vi "Draw Estimated Pose Covariance.vi"(10 "State Uncertainty":T1, 11 "Estimated State":T1) -> (3 "Covariance Ellipses":cluster{dbl[], dbl[]}[](graph))   [LabVIEW 2020]
uses:
  <vilib>/Analysis/Matrix/Datatypes/RealMatrix.ctl
  <vilib>/Analysis/baseanly.llb/Real A x B.vi
  <vilib>/Analysis/baseanly.llb/A x Vector.vi
  <vilib>/Analysis/7linalg.llb/Real SVD Decomposition.vi
  <vilib>/Analysis/Matrix/Numeric/Conversions/Matrix To Array - RM.vi
  <vilib>/Analysis/NI_AALPro.lvlib
  <vilib>/Analysis/NI_AALBase.lvlib
  <vilib>/Analysis/Matrix/NI_Matrix.lvlib
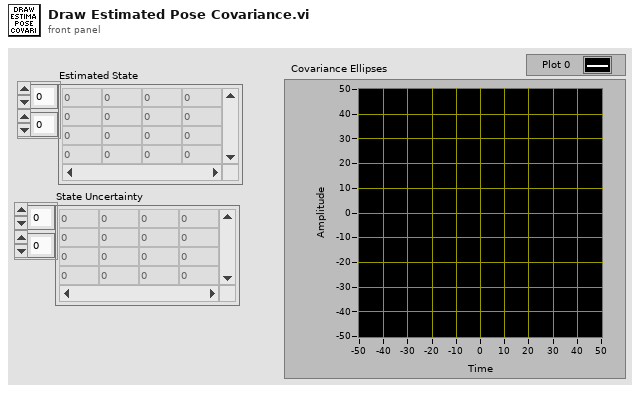
[diagram p1: front panel]
types:
  T1 = typedef "NI_Matrix.lvlib/RealMatrix.ctl" = dbl[][]
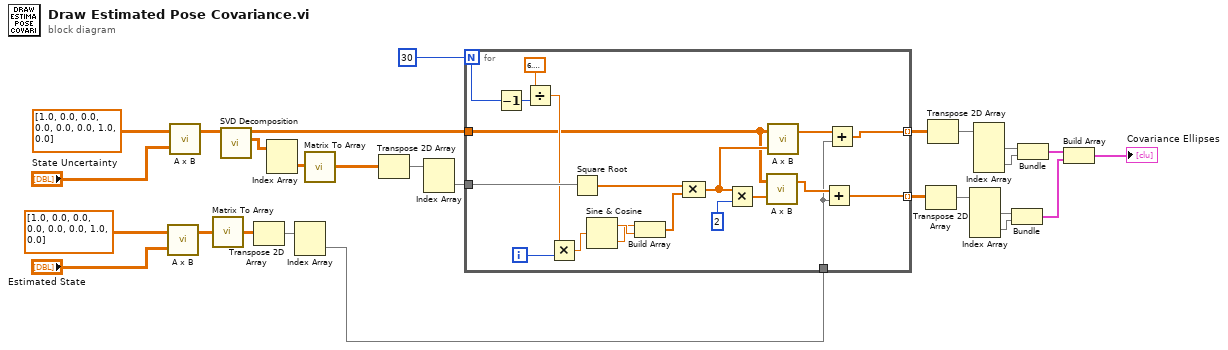
[diagram p0: block diagram]
diagram:
  n1 = call-poly <vilib>:"A x B.vi"("B"="Estimated State", "A"=T1 [[1.0, 0.0, 0.0, 0.0], [0.0, 0.0, 1.0, 0.0]] ("Initial Control Input")) -> ("A x B"=w4:T1)  [unwired: 1 out]
  n2 = call-poly <vilib>:"A x B.vi"("B"="State Uncertainty", "A"=T1 [[1.0, 0.0, 0.0, 0.0], [0.0, 0.0, 1.0, 0.0]] ("Initial Control Input")) -> ("A x B"=w23:T1)  [unwired: 1 out]
  n3 = call-poly <vilib>:"Matrix To Array.vi"("Real Matrix"=w4) -> ("Real 2D Array"=w3:dbl[][])
  n4 = call-poly <vilib>:"SVD Decomposition.vi"("A"=w23) -> ("Matrix S"=w25:T1, "Matrix U"=w27:T1)  [unwired: 6 in, 3 out]
  n5 = Transpose 2D Array(2D array=w3) -> (transposed array=w2:dbl[][])
  n6 = Index Array(array=w25) -> (element=w22:T1)  [unwired: 2 in]
  n7 = Index Array(array=w2) -> (element=w1:dbl[])  [unwired: 2 in]
  n8 = call-poly <vilib>:"Matrix To Array.vi"("Real Matrix"=w22) -> ("Real 2D Array"=w19:dbl[][])
  n9 = Transpose 2D Array(2D array=w19) -> (transposed array=w20:dbl[][])
  n10 = Index Array(array=w20) -> (element=w21:dbl[])  [unwired: 2 in]
  n11 = for {
    N: 30 -> [w37]
    tunnel: w27 -> [w33]
    tunnel: w21 -> [w47]
    tunnel: [w31] -> w18 mode=indexing
    tunnel: [w29] -> w14 mode=indexing
    tunnel: w1 -> [w28]
    i -> [w45]
    n12 = Decrement(x=w37) -> (x-1=w38:i32)
    n13 = Divide(x=6.283185307179586, y=w38) -> (x/y=w44:dbl)
    n14 = Multiply(x=w44, y=w45) -> (x*y=w43:dbl)
    n15 = Square Root(x=w47) -> (sqrt(x)=w40:dbl[])
    n16 = Sine & Cosine(0:w43) -> (1:w42:dbl, 2:w41:dbl)
    n17 = Build Array(w41, w42) -> (w39:dbl[])
    n18 = Compound Arithmetic op=MULTIPLY(w40, w39) -> (w36:dbl[])
    n19 = Multiply(x=w36, y=2) -> (x*y=w34:dbl[])
    n20 = call-poly <vilib>:"A x B.vi"("Vector"=w34, "A"=w33) -> ("A x Vector"=w30:dbl[])  [unwired: 1 out]
    n21 = call-poly <vilib>:"A x B.vi"("Vector"=w36, "A"=w33) -> ("A x Vector"=w32:dbl[])  [unwired: 1 out]
    n22 = Add(x=w30, y=w28) -> (x+y=w29:dbl[])
    n23 = Add(x=w32, y=w28) -> (x+y=w31:dbl[])
  }
  n24 = Transpose 2D Array(2D array=w14) -> (transposed array=w13:dbl[][])
  n25 = Transpose 2D Array(2D array=w18) -> (transposed array=w17:dbl[][])
  n26 = Index Array(array=w13) -> (element #1=w12:dbl[], element #2=w11:dbl[])  [unwired: 4 in]
  n27 = Index Array(array=w17) -> (element #1=w16:dbl[], element #2=w15:dbl[])  [unwired: 4 in]
  n28 = Bundle(w12, w11) -> (w9:cluster{dbl[], dbl[]})  [unwired: 1 in]
  n29 = Bundle(w16, w15) -> (w10:cluster{dbl[], dbl[]})  [unwired: 1 in]
  n30 = Build Array(w10, w9) -> (→"Covariance Ellipses":cluster{dbl[], dbl[]}[])
